vi "2delaypoints.vi"(2 "Offset (mm)":dbl, 3 "delay table [fs]":string[][](table)) -> (0 "delay points [mm]":dbl[](array[numeric]), 1 "delay pointss [fs]":dbl[](array[numeric]))   [LabVIEW 2020]
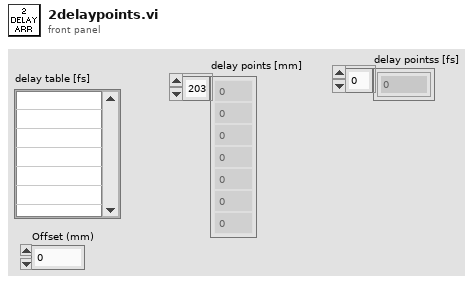
[diagram p1: front panel]
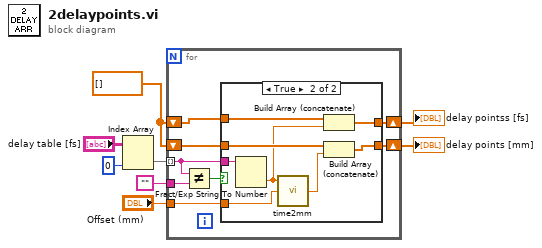
[diagram p0: block diagram]
diagram:
  w1 = dbl[] []
  n1 = Index Array(array="delay table [fs]", index (col)=0 ("disabled index (col)")) -> (element=w8:string[])  [unwired: 1 in]
  n2 = for {
    tunnel: w8 -> [w14] mode=indexing
    shift-right: [w16] -> w6
    shift-left: w1 -> [w15]
    tunnel: "" -> [w13]
    tunnel: "Offset (mm)" -> [w11]
    shift-right: [w10] -> w2
    shift-left: w1 -> [w9]
    n3 = Not Equal?(x=w14, y=w13) -> (x != y?=w12:bool)
    n4 = case shown="True" w12 {
      tunnel: w14 -> [_ w26]
      tunnel: [w18 w25] -> w16
      tunnel: w15 -> [w18 w24]
      tunnel: w11 -> [_ w22]
      tunnel: [w17 w20] -> w10
      tunnel: w9 -> [w17 w19]
      frame False {
      }
      frame True {
        n5 = Fract/Exp String To Number(string=w26) -> (number=w21:dbl)  [unwired: 3 in, 1 out]
        n6 = call "time2mm.vi"("Offset (mm)"=w22, "time"=w21) -> ("position (mm)"=w23:dbl)  [unwired: 1 in]
        n7 = Build Array (concatenate)(w19, w21) -> (w20:dbl[])
        n8 = Build Array (concatenate)(w24, w23) -> (w25:dbl[])
      }
    }
  }
  "delay points [mm]" <- w6
  "delay pointss [fs]" <- w2
